vi "WPI_GyroSetGain.vi"(8 "error in (no error)":errorcluster, 10 "Gain (VoltsPerDegree/Second)":dbl=0.0125, 11 "GyroDevRef":T1={"DevStatus"={"status"=FALSE, "code"=0, "source"=""}, "Analog Module"=enum."Analog Module 2", "Analog Channel"=enum."AI 1", "Offset"=0.0, "Gain (VoltsPerDegree/Second)"=0.0}) -> (0 "error out":errorcluster, 3 "GyroDevRef":T1={"DevStatus"={"status"=FALSE, "code"=0, "source"=""}, "Analog Module"=enum."Analog Module 2", "Analog Channel"=enum."AI 1", "Offset"=0.0, "Gain (VoltsPerDegree/Second)"=0.0})   [LabVIEW 2013]
doc: "Specifies the voltage used per degree of rotation per second. This VI specifies one of the parameters used by the GetAngle VI to calculate and report the heading of the robot.\n\nThis software is licensed. Open the labview\\readme\\WPI Robotics Library Open Source License.txt file for more information."
uses:
  <vilib>/Rock Robotics/WPI/Gyro/WPI_GyroDevRef.ctl
  <vilib>/Rock Robotics/SystemInterfaces/Typedef/FPGA_TypedefAnalogModule.ctl
  <vilib>/Rock Robotics/SystemInterfaces/AI/FPGA_AIChannel.ctl
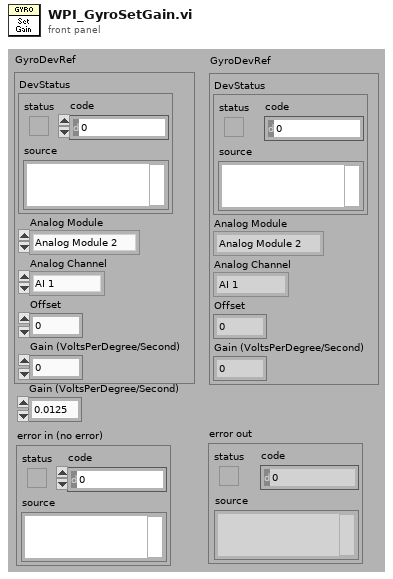
[diagram p1: front panel]
types:
  T1 = typedef "WPI_GyroDevRef.ctl" = cluster{"DevStatus":errorcluster, "Analog Module":T2, "Analog Channel":T3, "Offset":dbl, "Gain (VoltsPerDegree/Second)":dbl}
  T2 = typedef "FPGA_TypedefAnalogModule.ctl" = enum16{"Analog Module 1", "Analog Module 2"}
  T3 = typedef "FPGA_AIChannel.ctl" = enum8{"AI 1", "AI 2", "AI 3", "AI 4", "AI 5", "AI 6", "AI 7", "AI 8", "Invalid"}
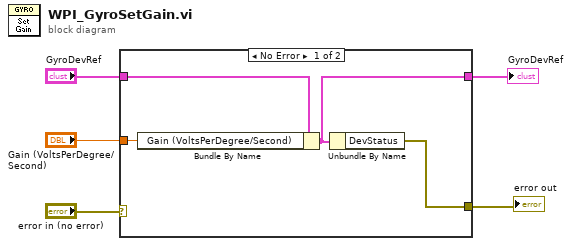
[diagram p0: block diagram]
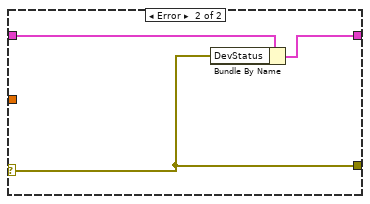
[diagram p2: hidden frame]
diagram:
  n1 = case shown="No Error" "error in (no error)" {
    selector: "error in (no error)" -> [_ w10]
    tunnel: "GyroDevRef" -> [w9 w12]
    tunnel: [w7 w11] -> w4
    tunnel: "Gain (VoltsPerDegree/Second)" -> [w8 _]
    tunnel: [w6 w10] -> w1
    frame No Error {
      n2 = Bundle By Name(cluster=w9, "Gain (VoltsPerDegree/Second)"=w8) -> (w7:T1)
      n3 = Unbundle By Name(w7) -> ("DevStatus"=w6:errorcluster)
    }
    frame Error {
      n4 = Bundle By Name(cluster=w12, "DevStatus"=w10) -> (w11:T1)
    }
  }
  "GyroDevRef" <- w4
  "error out" <- w1
